vi "Delete Data (Row).vi"(0 "Filepath":path, 5 "DataIndex":i32, 7 "StatIndex":i32, 9 "StatRows":i32, 11 "Error In":errorcluster) -> (15 "Error Out":errorcluster)   [LabVIEW 2013]
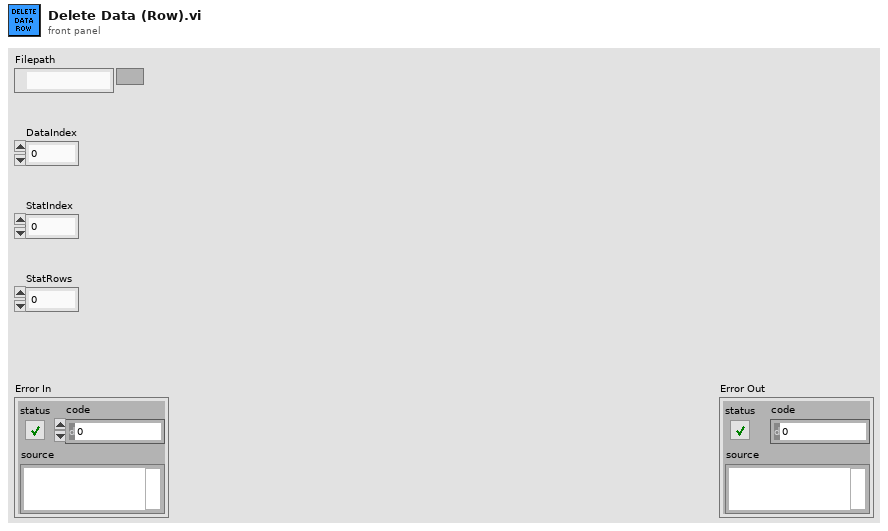
[diagram p1: front panel]
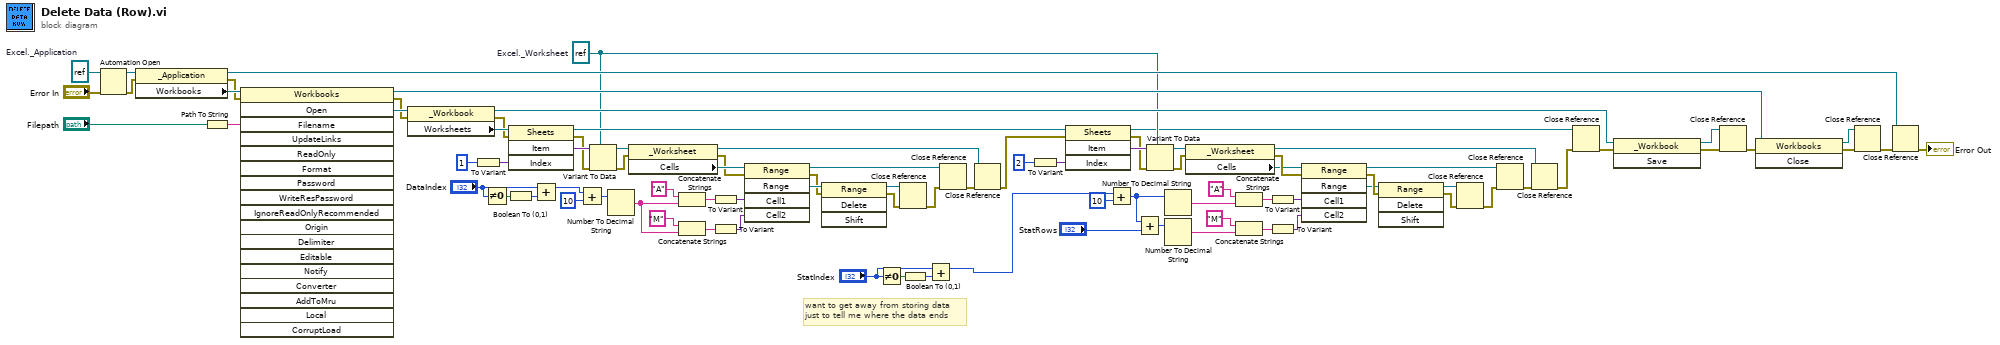
[diagram p0: block diagram]
diagram:
  w15 = refnum<k7> refnum  # Excel._Worksheet
  w84 = refnum<k7> refnum  # Excel._Application
  # "want to get away from storing data\njust to tell me where the data ends"
  n1 = Automation Open(error in (no error)="Error In", Automation Refnum=w84) -> (Automation Refnum=w85:refnum<k7>, error out=w86:errorcluster)  [unwired: 2 in]
  n2 = property class="_Application"(reference=w85, error in=w86) -> (reference out=w77:refnum<k7>, error out=w78:errorcluster, "Workbooks"=w87:refnum<k7>)
  n3 = Path To String(path="Filepath") -> (string=w74:string)
  n4 = invoke class="Workbooks" method="Open"(reference=w87, error in=w78, "Filename"=w74) -> (reference out=w81:refnum<k7>, error out=w76:errorcluster, "Open"=w83:refnum<k7>)  [unwired: 15 in, 15 out]
  n5 = property class="_Workbook"(reference=w83, error in=w76) -> (reference out=w70:refnum<k7>, error out=w57:errorcluster, "Worksheets"=w58:refnum<k7>)
  n6 = To Variant(anything=1) -> (Variant=w66:variant)
  n7 = Not Equal To 0?(x="DataIndex") -> (x != 0?=w7:bool)
  n8 = Boolean To (0,1)(Boolean=w7) -> (0, 1=w6:i16)
  n9 = invoke class="Sheets" method="Item"(reference=w58, error in=w57, "Index"=w66) -> (reference out=w16:refnum<k7>, error out=w64:errorcluster, "Item"=w65:variant)  [unwired: 1 in, 1 out]
  n10 = Add(x="DataIndex", y=w6) -> ()  [unwired: 1 out]
  n11 = Add(x="DataIndex", y=10) -> (x+y=w49:i32)
  n12 = Variant To Data(error in=w64, type=w15, Variant=w65) -> (data=w54:refnum<k7>, error out=w53:errorcluster)
  n13 = Number To Decimal String(number=w49) -> (decimal integer string=w44:string)  [unwired: 1 in]
  n14 = property class="_Worksheet"(reference=w54, error in=w53) -> (reference out=w62:refnum<k7>, error out=w55:errorcluster, "Cells"=w56:refnum<k7>)
  n15 = Concatenate Strings("A" ("ColumnIndex"), w44) -> (w42:string)
  n16 = Concatenate Strings("M" ("ColumnIndex"), w44) -> (w43:string)
  n17 = To Variant(anything=w42) -> (Variant=w59:variant)
  n18 = To Variant(anything=w43) -> (Variant=w51:variant)
  n19 = invoke class="Range" method="Range"(reference=w56, error in=w55, "Cell1"=w59, "Cell2"=w51) -> (reference out=w61:refnum<k7>, error out=w48:errorcluster, "Range"=w52:refnum<k7>)  [unwired: 1 in, 2 out]
  n20 = invoke class="Range" method="Delete"(reference=w52, error in=w48) -> (reference out=w47:refnum<k7>, error out=w46:errorcluster)  [unwired: 2 in, 2 out]
  n21 = Not Equal To 0?(x="StatIndex") -> (x != 0?=w4:bool)
  n22 = Close Reference(reference=w47, error in (no error)=w46) -> (error out=w45:errorcluster)
  n23 = Boolean To (0,1)(Boolean=w4) -> (0, 1=w5:i16)
  n24 = Add(x="StatIndex", y=w5) -> ()  [unwired: 1 out]
  n25 = Close Reference(reference=w61, error in (no error)=w45) -> (error out=w63:errorcluster)
  n26 = Close Reference(reference=w62, error in (no error)=w63) -> (error out=w14:errorcluster)
  n27 = To Variant(anything=2) -> (Variant=w17:variant)
  n28 = invoke class="Sheets" method="Item"(reference=w16, error in=w14, "Index"=w17) -> (reference out=w13:refnum<k7>, error out=w12:errorcluster, "Item"=w18:variant)  [unwired: 1 in, 1 out]
  n29 = Add(x="StatIndex", y=10) -> (x+y=w10:i32)
  n30 = Add(x=w10, y="StatRows") -> (x+y=w8:i32)
  n31 = Variant To Data(error in=w12, type=w15, Variant=w18) -> (data=w26:refnum<k7>, error out=w27:errorcluster)
  n32 = Number To Decimal String(number=w10) -> (decimal integer string=w35:string)  [unwired: 1 in]
  n33 = Number To Decimal String(number=w8) -> (decimal integer string=w9:string)  [unwired: 1 in]
  n34 = property class="_Worksheet"(reference=w26, error in=w27) -> (reference out=w20:refnum<k7>, error out=w25:errorcluster, "Cells"=w24:refnum<k7>)
  n35 = Concatenate Strings("A" ("ColumnIndex"), w35) -> (w37:string)
  n36 = Concatenate Strings("M" ("ColumnIndex"), w9) -> (w36:string)
  n37 = To Variant(anything=w37) -> (Variant=w23:variant)
  n38 = To Variant(anything=w36) -> (Variant=w29:variant)
  n39 = invoke class="Range" method="Range"(reference=w24, error in=w25, "Cell1"=w23, "Cell2"=w29) -> (reference out=w21:refnum<k7>, error out=w31:errorcluster, "Range"=w28:refnum<k7>)  [unwired: 1 in, 2 out]
  n40 = invoke class="Range" method="Delete"(reference=w28, error in=w31) -> (reference out=w32:refnum<k7>, error out=w33:errorcluster)  [unwired: 2 in, 2 out]
  n41 = Close Reference(reference=w32, error in (no error)=w33) -> (error out=w34:errorcluster)
  n42 = Close Reference(reference=w21, error in (no error)=w34) -> (error out=w19:errorcluster)
  n43 = Close Reference(reference=w20, error in (no error)=w19) -> (error out=w11:errorcluster)
  n44 = Close Reference(reference=w13, error in (no error)=w11) -> (error out=w75:errorcluster)
  n45 = invoke class="_Workbook" method="Save"(reference=w70, error in=w75) -> (reference out=w71:refnum<k7>, error out=w72:errorcluster)  [unwired: 1 in, 1 out]
  n46 = Close Reference(reference=w71, error in (no error)=w72) -> (error out=w73:errorcluster)
  n47 = invoke class="Workbooks" method="Close"(reference=w81, error in=w73) -> (reference out=w80:refnum<k7>, error out=w79:errorcluster)  [unwired: 1 in, 1 out]
  n48 = Close Reference(reference=w80, error in (no error)=w79) -> (error out=w82:errorcluster)
  n49 = Close Reference(reference=w77, error in (no error)=w82) -> (error out=→"Error Out":errorcluster)
